vi "KeyDown Event Callback.vi"(4 "DataGridView in":refnum<class "DataGridView.lvclass">, 5 "Event Data":cluster{"sender":refnum<k24>, "e":refnum<k24>}, 6 "Control Ref":refnum<k24>, 7 "Event Common Data":T1) -> ()   [LabVIEW 2016, in "DataGrid.lvlib" / "DataGridView.lvclass"]
doc: "This call back event captures any key press and returns it to the labview user event with key codes and modifies for keyboard detection."
uses:
  <userlib>/LabVIEWdotNetDataGrid/source/DataGridView/DataGridView.lvclass
  System.Windows.Forms
  <userlib>/LabVIEWdotNetDataGrid/source/Events/KeyDown/KeyDown.lvclass
  C:/Program Files (x86)/National Instruments/LabVIEW 2016/user.lib/LabVIEWdotNetDataGrid/source/Events/Abstract EVENT/Abstract EVENT.lvclass
  <userlib>/LabVIEWdotNetDataGrid/source/Events/KeyDown/KeyDown.lvclass/KeyDown.ctl
  <userlib>/LabVIEWdotNetDataGrid/source/Events/KeyDown/Write Alt.vi
  <userlib>/LabVIEWdotNetDataGrid/source/Events/KeyDown/Write Control.vi
  <userlib>/LabVIEWdotNetDataGrid/source/Events/KeyDown/Write KeyCode.vi
  <userlib>/LabVIEWdotNetDataGrid/source/Events/KeyDown/Write KeyData.vi
  <userlib>/LabVIEWdotNetDataGrid/source/Events/KeyDown/Write KeyValue.vi
  <userlib>/LabVIEWdotNetDataGrid/source/Events/KeyDown/Write Modifiers.vi
  <userlib>/LabVIEWdotNetDataGrid/source/Events/KeyDown/Write Shift.vi
panel:
  out "reference out":refnum<k24>
  in  "error in (no error)":errorcluster
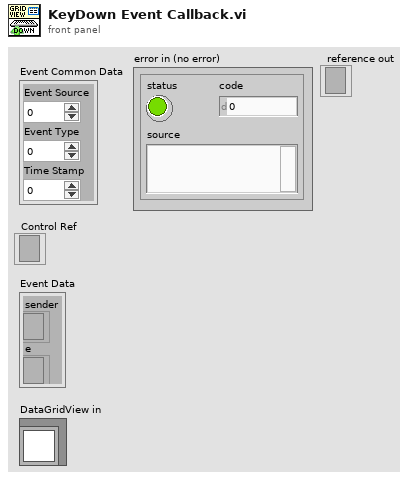
[diagram p1: front panel]
types:
  T1 = cluster{"Event Source":i32, "Event Type":u32, "Time Stamp":u32}
  T2 = cluster{"CellClicked":refnum<user-event>, "CellValue Changed":refnum<user-event>, "KeyDown":refnum<user-event>, "DataError":refnum<user-event>, "UserAddedRow":refnum<user-event>, "UserDeletedRow":refnum<user-event>}
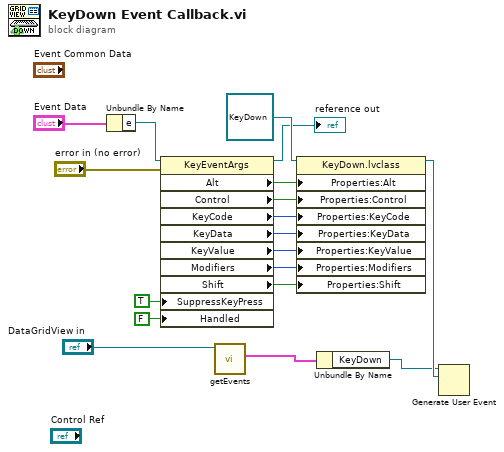
[diagram p0: block diagram]
diagram:
  n1 = Unbundle By Name("Event Data") -> ("e"=w18:refnum<k24>)
  n2 = property class="KeyEventArgs"(reference=w18, error in="error in (no error)", "SuppressKeyPress"=TRUE, "Handled"=FALSE) -> (reference out=→"reference out":refnum<k24>, "Alt"=w9:bool, "Control"=w8:bool, "KeyCode"=w7:i32, "KeyData"=w6:i32, "KeyValue"=w5:i32, "Modifiers"=w4:i32, "Shift"=w3:bool)  [unwired: 1 out]
  n3 = call <userlib>:"getEvents.vi"("DataGridView in"="DataGridView in") -> ("userEvents"=w14:T2)  [unwired: 8 in, 2 out]
  n4 = property class="KeyDown.lvclass"(reference=refnum<class "KeyDown.lvclass"> refnum ("DataGrid.lvlib:KeyPressed.lvclass"), "Properties:Alt"=w9, "Properties:Control"=w8, "Properties:KeyCode"=w7, "Properties:KeyData"=w6, "Properties:KeyValue"=w5, "Properties:Modifiers"=w4, "Properties:Shift"=w3) -> (reference out=w15:refnum<class "KeyDown.lvclass">)  [unwired: 1 in, 1 out]
  n5 = Unbundle By Name(w14) -> ("KeyDown"=w13:refnum<user-event>)
  n6 = Generate User Event(user event=w13, event data cluster=w15) -> ()  [unwired: 2 in, 2 out]
